vi "Run Test Case.vi"(8 "error in (no error)":errorcluster, 10 "Test Case":refnum<class "LUnit Test Case.lvclass">, 11 "Slave Test Runner In":refnum<class "Slave Test Runner.lvclass">) -> (0 "error out":errorcluster, 3 "Slave Test Runner Out":refnum<class "Slave Test Runner.lvclass">)   [LabVIEW 2020, in "Slave Test Runner.lvclass"]
uses:
  Slave Test Runner.lvclass
  C:/Users/anton/Documents/GitHub/LUnit/source/Application Framework/Process Classes/Process/Process.lvclass
  Test Case/LUnit Test Case.lvclass
  Application Framework/Process Classes/Process/Process.lvclass/Process.ctl
  Application Framework/Process Classes/Process/Process.lvclass
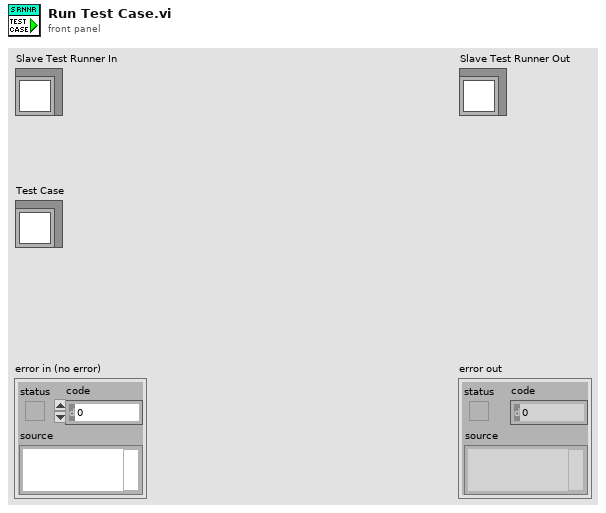
[diagram p1: front panel]
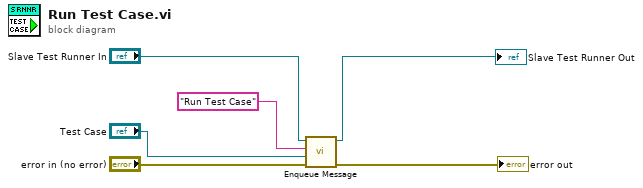
[diagram p0: block diagram]
diagram:
  n1 = call "Enqueue Message.vi"("error in (no error)"="error in (no error)", "Message Data"="Test Case", "Message"="Run Test Case", "Process In"="Slave Test Runner In") -> ("error out"=→"error out":errorcluster, "Process Out"=→"Slave Test Runner Out":refnum<class "Slave Test Runner.lvclass">)  [unwired: 6 in]
